vi "GVmotor_format_data.vi"(9 "analog":dbl, 10 "turn":dbl, 11 "time":timestamp) -> (3 "waveform_array":waveform(dbl)[](array[waveform]))   [LabVIEW 2019]
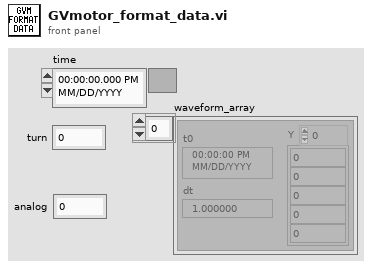
[diagram p1: front panel]
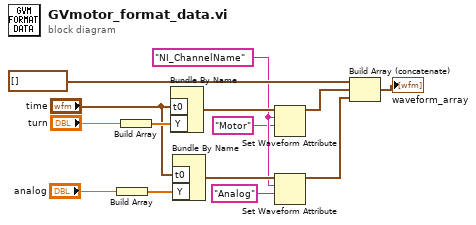
[diagram p0: block diagram]
diagram:
  w5 = "NI_ChannelName" ("name")
  n1 = Build Array("analog") -> (w8:dbl[])
  n2 = Build Array("turn") -> (w13:dbl[])
  n3 = Bundle By Name("t0"="time", "Y"=w13) -> (w7:waveform(dbl))  [unwired: 1 in]
  n4 = Bundle By Name("t0"="time", "Y"=w8) -> (w6:waveform(dbl))  [unwired: 1 in]
  n5 = Set Waveform Attribute(5:"Motor", 6:w5, 7:w7) -> (3:w2:waveform(dbl))  [unwired: 1 in, 2 out]
  n6 = Set Waveform Attribute(5:"Analog", 6:w5, 7:w6) -> (3:w1:waveform(dbl))  [unwired: 1 in, 2 out]
  n7 = Build Array (concatenate)(waveform(dbl)[] [], w2, w1) -> (→"waveform_array":waveform(dbl)[])
